vi "subSave_AquireTimeInformation.vi"() -> (0 "time out":string)   [LabVIEW 2015]
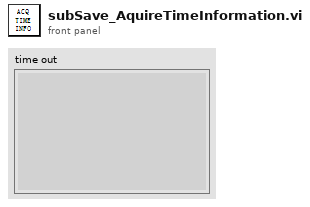
[diagram p1: front panel]
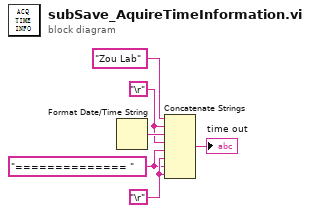
[diagram p0: block diagram]
diagram:
  w2 = "\r"
  w1 = "============== " ("string")
  w4 = "\r"
  n1 = Format Date/Time String() -> (date/time string=w6:string)  [unwired: 3 in]
  n2 = Concatenate Strings("Zou Lab" ("string"), w4, w6, w4, w1, w2, w1, w2) -> (→"time out":string)
